vi "Decode Application Message (Type).vi"(7 "Type":variant, 8 "error in (no error)":errorcluster, 10 "PUBLISH":refnum<class "PUBLISH.lvclass">, 11 "Client in":refnum<class "Client.lvclass">) -> (0 "error out":errorcluster, 1 "Payload":variant, 2 "Topic":string, 3 "Client out":refnum<class "Client.lvclass">)   [LabVIEW 2013, in "MQTT Client.lvlib" / "Client.lvclass"]
uses:
  Client.lvclass
  <vilib>/LabVIEW Open Source Project/MQTT Control Packets/Control Packets/PUBLISH/PUBLISH.lvclass
  <vilib>/LabVIEW Open Source Project/MQTT Connection/MQTT_Base/Base Class/MQTT_Base.lvclass
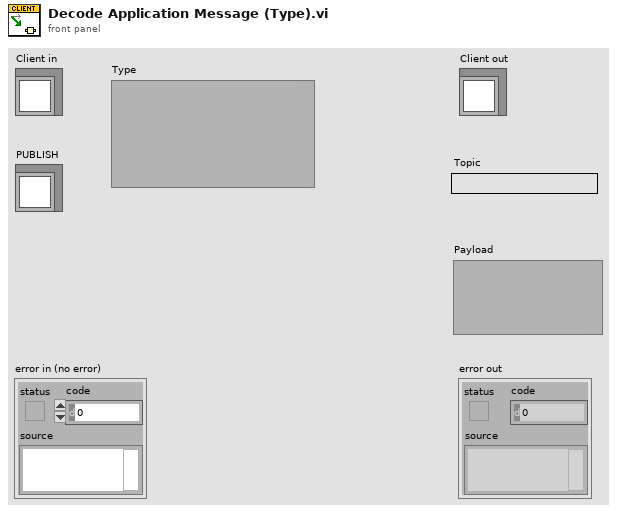
[diagram p1: front panel]
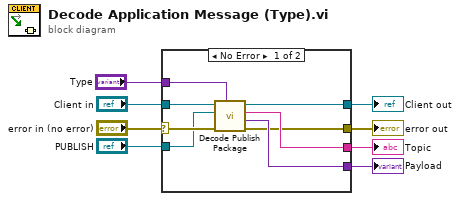
[diagram p0: block diagram]
diagram:
  n1 = case shown="No Error" "error in (no error)" {
    selector: "error in (no error)" -> [w10 w18]
    tunnel: [w11 w18] -> w7
    tunnel: [w16 w17] -> w5
    tunnel: "Client in" -> [w15 w17]
    tunnel: "PUBLISH" -> [w9 _]
    tunnel: [w12 _] -> w2
    tunnel: [w13 _] -> w3
    tunnel: "Type" -> [w14 _]
    frame No Error {
      n2 = call <vilib>:"Decode Publish Package.vi"("Type"=w14, "error in (no error)"=w10, "PUBLISH"=w9, "MQTT_Base in"=w15) -> ("error out"=w11:errorcluster, "Payload"=w12:variant, "Topic"=w13:string, "MQTT_Base out"=w16:refnum<class "Client.lvclass">)  [unwired: 4 in]
    }
    frame Error {
    }
  }
  "error out" <- w7
  "Client out" <- w5
  "Topic" <- w3
  "Payload" <- w2
